vi "Configure Null.vi"(0 "VISA resource name":refnum<visa-resource-name>, 1 "Channel (1: Channel 1)":u16(ring)=1 items=["Channel 1"=1, "Channel 2"=2], 5 "Function (0: Voltage)":u16(ring) items=["Voltage", "2-Wire Resistance", "4-Wire Resistance", "Temperature"], 7 "Null Mode (0: On)":u16(ring) items=["On", "Off", "Once"], 9 "Null Value (1.0)":dbl=1.0, 11 "error in (no error)":errorcluster) -> (4 "VISA resource name out":refnum<visa-resource-name>, 15 "error out":errorcluster)   [LabVIEW 2021, in "Agilent 34420.lvlib"]
doc: "Configures the null settings to negate the effects of long leads or additional impedences for more accurate measurements."
uses:
  <instrlib>/Agilent 34420/Agilent 34420.lvlib
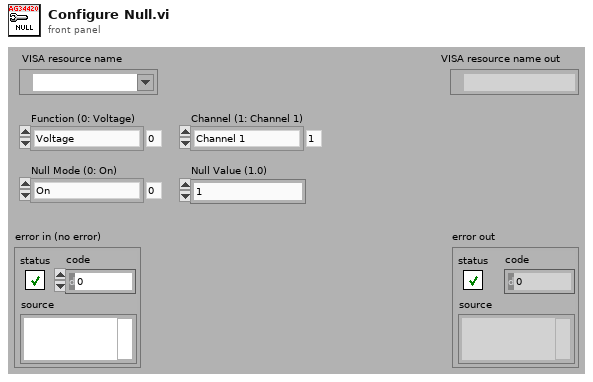
[diagram p1: front panel]
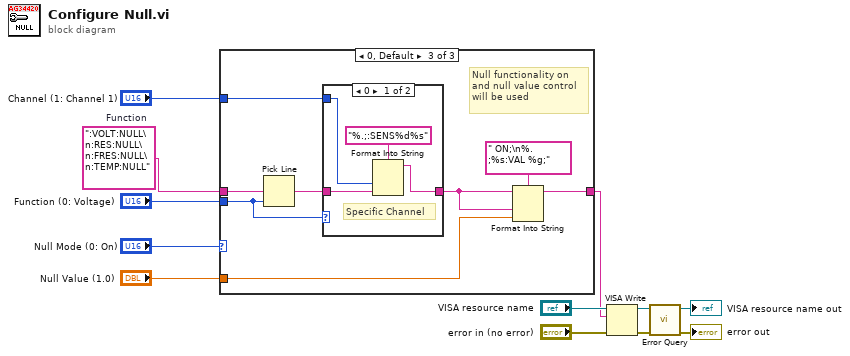
[diagram p0: block diagram]
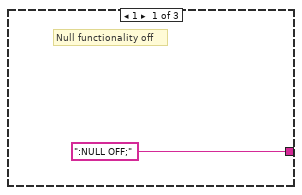
[diagram p2: hidden frame]
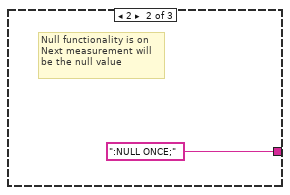
[diagram p3: hidden frame]
diagram:
  w8 = ":VOLT:NULL\n:RES:NULL\n:FRES:NULL\n:TEMP:NULL"  # Function
  n1 = case shown="0, Default" "Null Mode (0: On)" {
    tunnel: w8 -> [_ _ w22]
    tunnel: "Function (0: Voltage)" -> [_ _ w21]
    tunnel: "Channel (1: Channel 1)" -> [_ _ w20]
    tunnel: "Null Value (1.0)" -> [_ _ w16]
    tunnel: [":NULL OFF;" ":NULL ONCE;" w15] -> w1
    frame 1 {
      # "Null functionality off"
    }
    frame 2 {
      # "Null functionality is on\nNext measurement will\nbe the null value"
    }
    frame 0, Default {
      # "Null functionality on\nand null value control\nwill be used"
      n2 = Pick Line(multi-line string=w22, line index=w21) -> (output string=w19:string)  [unwired: 1 in]
      n3 = case shown="0" w21 {
        tunnel: w20 -> [w26 _]
        tunnel: w19 -> [w24 w27]
        tunnel: [w23 w27] -> w17
        frame 0 {
          # "Specific Channel"
          n4 = Format Into String(format string="%.;:SENS%d%s", w26, w24) -> (resulting string=w23:string)  [unwired: 2 in, 1 out]
        }
        frame 1, Default {
          # "No channel\nnecessary"
        }
      }
      n5 = Format Into String(format string=" ON;\n%.;%s:VAL %g;", initial string=w17, w17, w16) -> (resulting string=w15:string)  [unwired: 1 in, 1 out]
    }
  }
  n6 = VISA Write(VISA resource name="VISA resource name", write buffer=w1, error in (no error)="error in (no error)") -> (VISA resource name out=w7:refnum<visa-resource-name>, error out=w6:errorcluster)  [unwired: 1 out]
  n7 = call <instrlib>:"Error Query.vi"("error in (no error)"=w6, "VISA resource name"=w7) -> ("error out"=→"error out":errorcluster, "VISA resource name out"=→"VISA resource name out":refnum<visa-resource-name>)  [unwired: 6 in, 2 out]
